vi "T3AWG Gen Wave.vi"(0 "f [Hz]":dbl, 1 "A-dither [V]":dbl, 2 "t3awg":T1={"VISA"="", "use ext ref"=FALSE, "ext ref [Hz]"=0.0, "load Z"=enum."High Z", "ramdac max n"=0, "noise dither [V]"=0.0, "t3awg fs rules"=[], "channels"=0, "ramdac min n"=0, "channel list"=[], "gen resl [Vpp]"=0.0, "wave data format"=enum."Binary"} {"t3awg fs rules"."fs-step [Hz]" format="%#_6p"; "t3awg fs rules"."fs-max [Hz]" format="%#_6p"; "t3awg fs rules"."for f0 <" format="%#_6p"; "t3awg fs rules"."fs-min [Hz]" format="%#_6p"}, 3 "exact setup (True)":bool=TRUE, 5 "fs [Hz]":dbl, 7 "phi [rad]":dbl, 9 "N":i32, 11 "A [V]":dbl, 12 "gen A-max [V]":dbl=3.0, 13 "gen A-resl [V]":dbl=0.001) -> (4 "wave":dbl[](array[numeric]), 6 "gen amp to set [V]":dbl, 10 "f real [Hz]":dbl, 14 "N out":i32, 15 "f real error [-]":dbl)   [LabVIEW 2020, in "Active Technologies AWG3000.lvlib"]
uses:
  Active Technologies AWG3000.lvlib
  T3AWG Session.ctl
  T3AWG Load Z.ctl
  fgen_ramdac_fs_rules.ctl
  T3AWG Channel.ctl
panel:
  out "generator step [V]":dbl
  out "min value":dbl
  out "max value":dbl
  out "Waveform Graph":dbl[](graph)
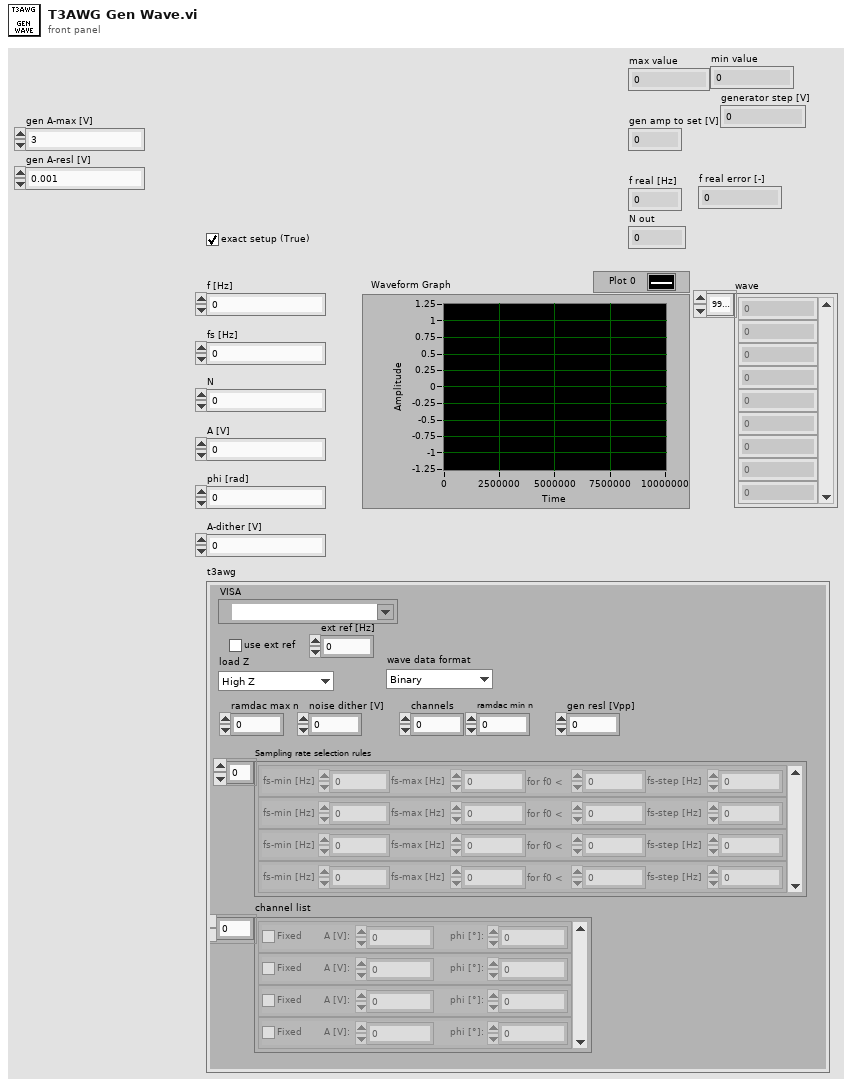
[diagram p1: front panel]
types:
  T1 = typedef "Active Technologies AWG3000.lvlib/T3AWG Session.ctl" = cluster{"VISA":refnum<visa-resource-name>, "use ext ref":bool, "ext ref [Hz]":dbl, "load Z":T2, "ramdac max n":i32, "noise dither [V]":dbl, "t3awg fs rules":T3[], "channels":i32, "ramdac min n":i32, "channel list":T4[], "gen resl [Vpp]":dbl, "wave data format":T5}
  T2 = typedef "Active Technologies AWG3000.lvlib/T3AWG Load Z.ctl" = enum16{"High Z", "50 Ohm"}
  T3 = typedef "Active Technologies AWG3000.lvlib/fgen_ramdac_fs_rules.ctl" = cluster{"fs-min [Hz]":dbl, "fs-max [Hz]":dbl, "for f0 < ":dbl, "fs-step [Hz]":dbl}
  T4 = typedef "Active Technologies AWG3000.lvlib/T3AWG Channel.ctl" = cluster{"Fixed":bool, "A [V]:":dbl, "phi [°]:":dbl}
  T5 = typedef "Active Technologies AWG3000.lvlib/T3AWG Wave Format" = enum16{"Text", "Binary"}
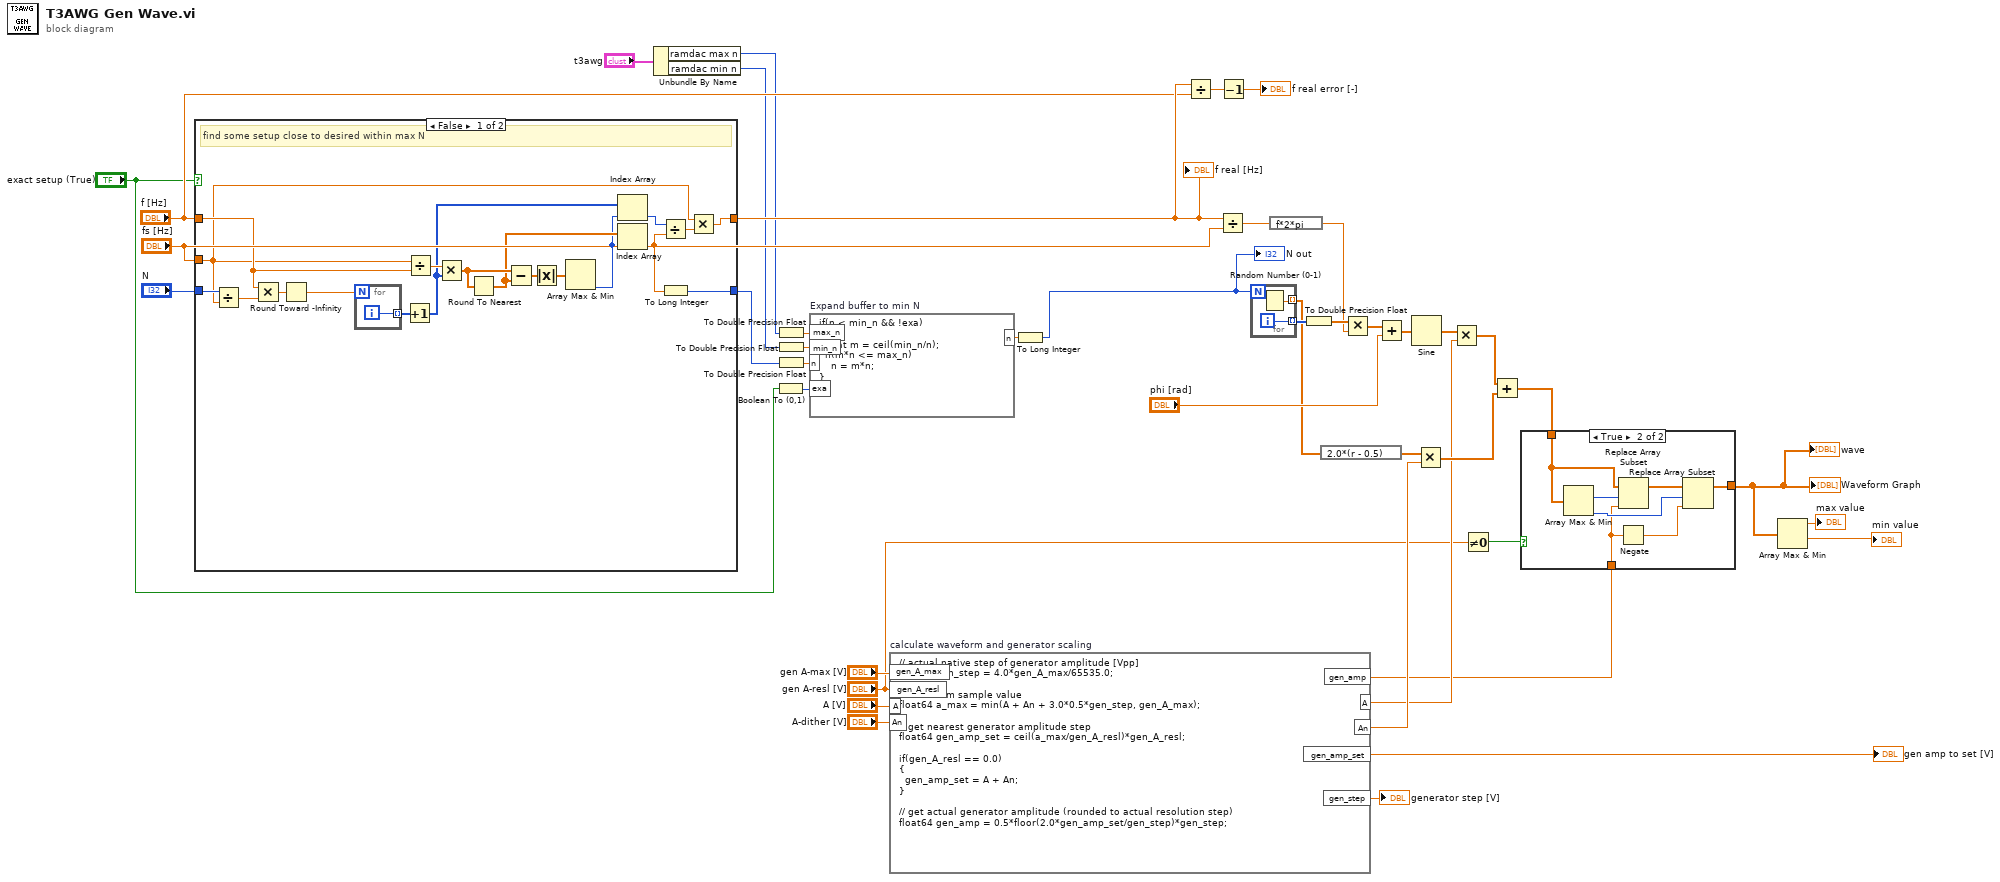
[diagram p0: block diagram]
diagram:
  n1 = case shown="False" "exact setup (True)" {
    tunnel: [w46 w65] -> w20
    tunnel: "N" -> [w62 w65]
    tunnel: [w45 w64] -> w29
    tunnel: "f [Hz]" -> [w58 w64]
    tunnel: "fs [Hz]" -> [w48 _]
    frame False {
      # "find some setup close to desired within max N"
      n2 = Divide(x=w62, y=w48) -> (x/y=w61:dbl)
      n3 = Multiply(x=w58, y=w61) -> (x*y=w60:dbl)
      n4 = Round Toward -Infinity(1:w60) -> (0:w44:dbl)
      n5 = for {
        N: w44 -> [_]
        tunnel: [w63] -> w59 mode=indexing
        i -> [w63]
      }
      n6 = Increment(x=w59) -> (x+1=w53:i32[])
      n7 = Divide(x=w48, y=w58) -> (x/y=w57:dbl)
      n8 = Multiply(x=w57, y=w53) -> (x*y=w56:dbl[])
      n9 = Round To Nearest(number=w56) -> (nearest integer value=w52:dbl[])
      n10 = Subtract(x=w56, y=w52) -> (x-y=w55:dbl[])
      n11 = Absolute Value(x=w55) -> (abs(x)=w54:dbl[])
      n12 = Array Max & Min(array=w54) -> (min index (indices)=w51:i32)  [unwired: 3 out]
      n13 = Index Array(array=w53, index=w51) -> (element=w50:i32)
      n14 = Index Array(array=w52, index=w51) -> (element=w47:dbl)
      n15 = Divide(x=w50, y=w47) -> (x/y=w49:dbl)
      n16 = To Long Integer(number=w47) -> (32bit integer=w46:i32)
      n17 = Multiply(x=w48, y=w49) -> (x*y=w45:dbl)
    }
    frame True {
    }
  }
  "f real [Hz]" <- w29
  n18 = Unbundle By Name("t3awg") -> ("ramdac max n"=w18:i32, "ramdac min n"=w17:i32)
  n19 = Boolean To (0,1)(Boolean="exact setup (True)") -> (0, 1=w16:i16)
  n20 = To Double Precision Float(number=w18) -> (double precision float=w25:dbl)
  n21 = To Double Precision Float(number=w17) -> (double precision float=w24:dbl)
  n22 = To Double Precision Float(number=w20) -> (double precision float=w23:dbl)
  n23 = formula code="if(n < min_n && !exa)\n{\n  float m = ceil(min_n/n);\n  if(m*n <= max_n)\n    n = m*n;\n}" "Expand buffer to min N"("max_n"=w25, "min_n"=w24, "n"=w23, "exa"=w16) -> ("n"=w22:dbl)
  n24 = formula code="// actual native step of generator amplitude [Vpp]\nfloat64 gen_step = 4.0*gen_A_max/65535.0;\n\n// maximum sample value\nfloat64 a_max = min(A + An + 3.0*0.5*gen_step, gen_A_max);\n\n// get nearest generator amplitude step\nfloat64 gen_amp_set = ceil(a_max/gen_A_resl)*gen_A_resl;\n\nif(gen_A_resl == 0.0)\n{\n  gen_amp_set = A + An;\n}\n\n// get actual generator amplitude (rounded to actual resolution step)\nfloat64 gen_amp = 0.5*floor(2.0*gen_amp_set/gen_step)*gen_step;" "calculate waveform and generator scaling"("gen_A_max"="gen A-max [V]", "gen_A_resl"="gen A-resl [V]", "A"="A [V]", "An"="A-dither [V]") -> ("gen_amp"=w8:dbl, "A"=w10:dbl, "An"=w11:dbl, "gen_amp_set"=→"gen amp to set [V]":dbl, "gen_step"=→"generator step [V]":dbl)
  n25 = To Long Integer(number=w22) -> (32bit integer=w21:i32)
  "N out" <- w21
  n26 = Divide(x=w29, y="f [Hz]") -> (x/y=w27:dbl)
  n27 = Divide(x=w29, y="fs [Hz]") -> (x/y=w41:dbl)
  n28 = Decrement(x=w27) -> (x-1=→"f real error [-]":dbl)
  n29 = for {
    N: w21 -> [_]
    tunnel: [w67] -> w43 mode=indexing
    tunnel: [w66] -> w35 mode=indexing
    i -> [w67]
    n30 = Random Number (0-1)() -> (number: 0 to 1=w66:dbl)
  }
  n31 = expression code="f*2*pi"(w41) -> (w40:dbl)
  n32 = To Double Precision Float(number=w43) -> (double precision float=w42:dbl[])
  n33 = expression code="2.0*(r - 0.5)"(w35) -> (w34:dbl[])
  n34 = Multiply(x=w42, y=w40) -> (x*y=w39:dbl[])
  n35 = Add(x=w39, y="phi [rad]") -> (x+y=w37:dbl[])
  n36 = Sine(x=w37) -> (sin(x)=w36:dbl[])
  n37 = Multiply(x=w34, y=w11) -> (x*y=w32:dbl[])
  n38 = Multiply(x=w36, y=w10) -> (x*y=w33:dbl[])
  n39 = Not Equal To 0?(x="gen A-resl [V]") -> (x != 0?=w1:bool)
  n40 = Add(x=w33, y=w32) -> (x+y=w9:dbl[])
  n41 = case shown="True" w1 {
    tunnel: w9 -> [w68 w75]
    tunnel: w8 -> [_ w71]
    tunnel: [w68 w69] -> w7
    frame False {
    }
    frame True {
      n42 = Array Max & Min(array=w75) -> (max index (indices)=w74:i32, min index (indices)=w72:i32)  [unwired: 2 out]
      n43 = Replace Array Subset(array=w75, new element=w71, index=w74) -> (w73:dbl[])
      n44 = Negate(x=w71) -> (-x=w70:dbl)
      n45 = Replace Array Subset(array=w73, new element=w70, index=w72) -> (w69:dbl[])
    }
  }
  "wave" <- w7
  "Waveform Graph" <- w7
  n46 = Array Max & Min(array=w7) -> (max value=→"max value":dbl, min value=→"min value":dbl)  [unwired: 2 out]
